vi "EnumToRIng.vi"(11 "Enum":variant) -> (3 "Ring (Value)":u16)   [LabVIEW 2011]
uses:
  LVStringsAndValuesArrayTypeDef.ctl
panel:
  out "Enum Name":string
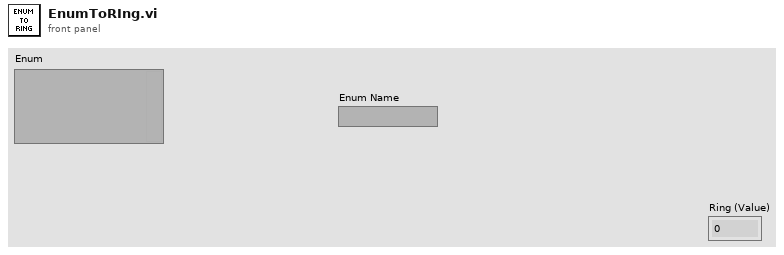
[diagram p1: front panel]
types:
  T1 = typedef "LVStringsAndValuesArrayTypeDef.ctl" = cluster{"String":string, "Value":ext}[]
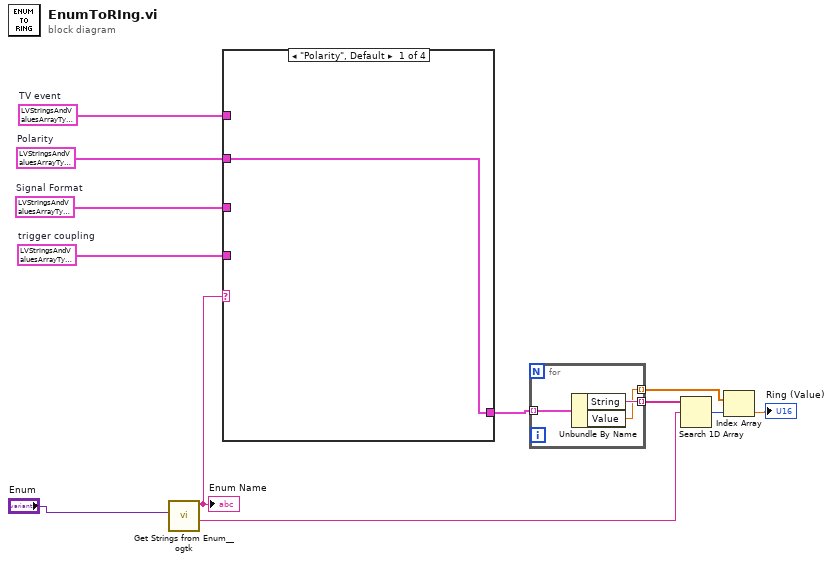
[diagram p0: block diagram]
diagram:
  w6 = T1 [{"String"="M-NTSC", "Value"=1.0}, {"String"="B/G-PAL", "Value"=2.0}, {"String"="SECAM", "Value"=3.0}, {"String"="M-PAL", "Value"=1001.0}, {"String"="480i/59.94 fps", "Value"=1010.0}, {"String"="480i/60 fps", "Value"=1011.0}, {"String"="480p/59.94 Fps", "Value"=1015.0}, {"String"="480p/60 Fps", "Value"=1016.0}, {"String"="576i/50 fps", "Value"=1020.0}, {"String"="576p/50 Fps", "Value"=1025.0}, {"String"="720p/50 Fps", "Value"=1031.0}, {"String"="720p/59.94 Fps", "Value"=1032.0}, {"String"="720p/60 Fps", "Value"=1033.0}, {"String"="1080i/50 fps", "Value"=1040.0}, {"String"="1080i/59.94 fps", "Value"=1041.0}, {"String"="1080i/60 fps", "Value"=1042.0}, {"String"="1080p/24 Fps", "Value"=1045.0}]  # Signal Format
  w3 = T1 [{"String"="Field 1", "Value"=1.0}, {"String"="Field 2", "Value"=2.0}, {"String"="Any Field", "Value"=3.0}, {"String"="Any Line", "Value"=4.0}, {"String"="Line Number", "Value"=5.0}]  # TV event
  w4 = T1 [{"String"="Positive", "Value"=1.0}, {"String"="Negative", "Value"=2.0}]  # Polarity
  w2 = T1 [{"String"="AC", "Value"=0.0}, {"String"="DC", "Value"=1.0}, {"String"="HF Reject", "Value"=3.0}, {"String"="LF Reject", "Value"=4.0}, {"String"="AC Plus HF Reject", "Value"=1001.0}]  # trigger coupling
  n1 = call "Get Strings from Enum__ogtk.vi"("Enum"="Enum") -> ("String Value"=w11:string, "Enum Name"=w7:string)  [unwired: 7 in, 2 out]
  "Enum Name" <- w7
  n2 = case shown="\"Polarity\", Default" w7 {
    tunnel: w6 -> [_ _ _ w16]
    tunnel: [w13 w14 w15 w16] -> w5
    tunnel: w4 -> [w13 _ _ _]
    tunnel: w3 -> [_ w14 _ _]
    tunnel: w2 -> [_ _ w15 _]
    frame "Polarity", Default {
    }
    frame "TV Event" {
    }
    frame "Coupling" {
    }
    frame "Signal Format" {
    }
  }
  n3 = for {
    tunnel: w5 -> [w19] mode=indexing
    tunnel: [w18] -> w12 mode=indexing
    tunnel: [w17] -> w10 mode=indexing
    n4 = Unbundle By Name(w19) -> ("String"=w18:string, "Value"=w17:ext)
  }
  n5 = Search 1D Array(1D array=w12, element=w11) -> (index of element=w9:i32)  [unwired: 1 in]
  n6 = Index Array(array=w10, index=w9) -> (element=→"Ring (Value)":ext)
